vi "TCP设备参数设置.vi"(8 "布尔文本.文本":string, 9 "section (optional)":string, 10 "监测项描述":string) -> (2 "布尔":bool=TRUE, 3 "输出簇":T1)   [LabVIEW 2016, in "环境动力监测库.lvlib"]
uses:
  <vilib>/Utility/miscctls.llb/LVPointTypeDef.ctl
  <vilib>/Utility/config.llb/NI_LVConfig.lvlib
panel:
  in  "Port:":string
  in  "data bits":u64=8 caption="数据比特" min=5 max=8 step=1
  in  "波特率":u64=19200
  in  "停止位":u16(ring)=10 items=["1.0"=10, "1.5"=15, "2.0"=20]
  in  "奇偶校验":u16(ring) items=["None", "Odd", "Even", "Mark", "Space"]
  in  "传感器型号:":string(combo)
  in  "输入簇":T1
  in  "站号":u64
  in  "返回":bool
  in  "增加":bool
  in  "IP address:":string
  in  "监测项描述:":string
  # "基本设置"
  # "如:红外XX"
  # "传感器选择"
  # "地址选择"
  # "站号配置"
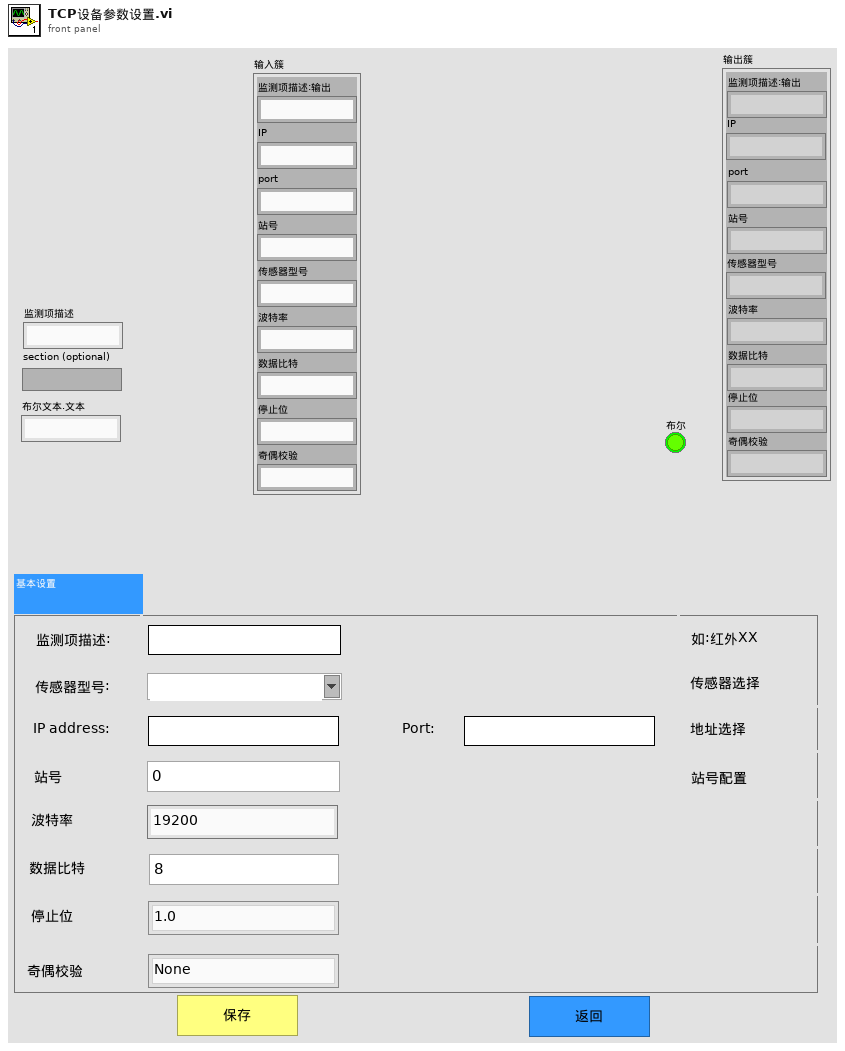
[diagram p1: front panel]
types:
  T1 = cluster{"监测项描述:输出":string, "IP":string, "port":string, "站号":string, "传感器型号":string, "波特率":string, "数据比特":string, "停止位":string, "奇偶校验":string}
  T2 = typedef "LVPointTypeDef.ctl" = cluster{"Horizontal":i16, "Vertical":i16}
  T3 = typedef "NI_LVConfig.lvlib/Config Data RefNum.ctl" = refnum<k1>
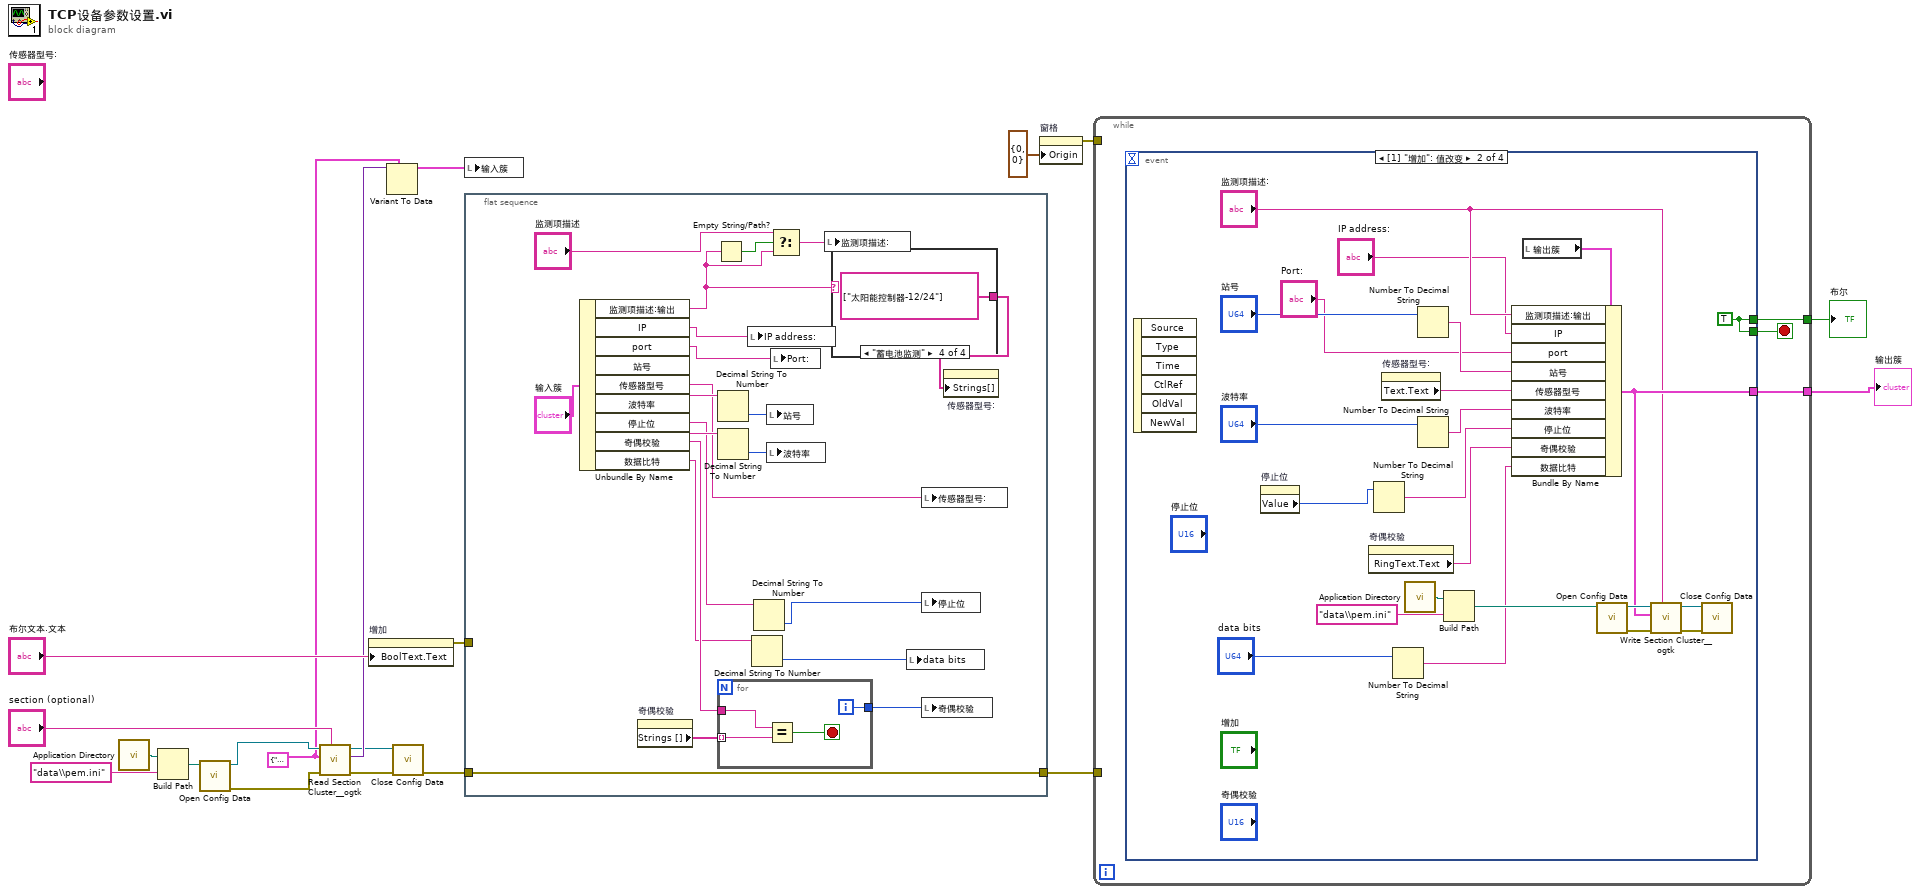
[diagram p0: block diagram]
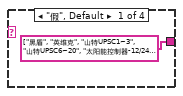
[diagram p2: hidden frame]
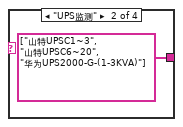
[diagram p3: hidden frame]
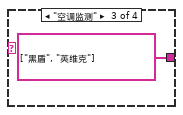
[diagram p4: hidden frame]
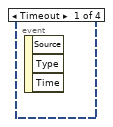
[diagram p5: hidden frame]
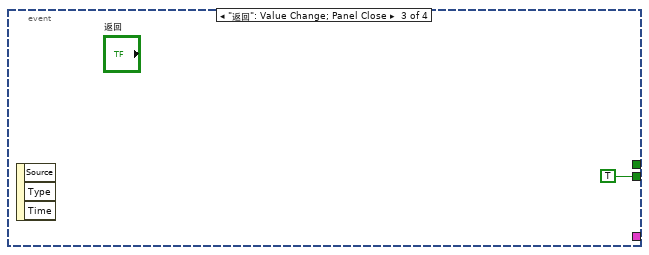
[diagram p6: hidden frame]
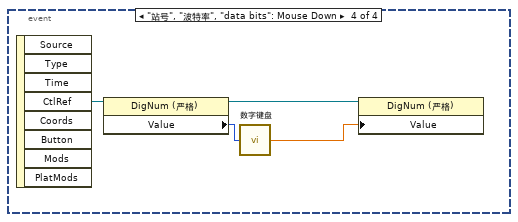
[diagram p7: hidden frame]
diagram:
  w1 = T1 {"监测项描述:输出"="", "IP"="", "port"="", "站号"="", "传感器型号"="", "波特率"="", "数据比特"="", "停止位"="", "奇偶校验"=""} ("数据")
  n1 = call <vilib>:"Application Directory.vi"() -> ("Application Directory"=w12:path)
  n2 = Build Path(base path=w12, name or relative path="data\\pem.ini" ("名称或相对路径")) -> (appended path=w13:path)
  n3 = call <vilib>:"Open Config Data.vi"("configuration file path"=w13) -> ("error out"=w14:errorcluster, "refnum"=w15:T3)  [unwired: 8 in, 1 out]
  n4 = call <userlib>:"Read Section Cluster__ogtk.vi"("section (optional)"="section (optional)", "error in (no error)"=w14, "Section Formatted Cluster Type"=w1, "refnum"=w15) -> ("error out"=w6:errorcluster, "Section Formatted Cluster"=w9:variant, "dup refnum"=w7:T3)  [unwired: 3 in, 2 out]
  n5 = property on="增加" class="Bool"("BoolText.Text"="布尔文本.文本") -> (error out=w5:errorcluster)  [unwired: 2 in, 1 out]
  n6 = Variant To Data(type=w1, Variant=w9) -> (data=w8:T1)  [unwired: 1 in, 1 out]
  n7 = call <vilib>:"Close Config Data.vi"("error in (no error)"=w6, "refnum"=w7) -> ("error out"=w4:errorcluster)  [unwired: 8 in, 1 out]
  n8 = local write "输入簇"(w8) -> ()
  n9 = flat-sequence {
    tunnel: w5 -> [_]
    tunnel: w4 -> [w38]
    tunnel: [w38] -> w3
    frame #0 {
      n10 = Unbundle By Name("输入簇") -> ("监测项描述:输出"=w21:string, "IP"=w24:string, "port"=w23:string, "站号"=w39:string, "传感器型号"=w22:string, "波特率"=w32:string, "停止位"=w28:string, "奇偶校验"=w29:string, "数据比特"=w26:string)
      n11 = property on="奇偶校验" class="Ring (严格)"() -> ("Strings []"=w30:string[])  [unwired: 2 in, 2 out]
      n12 = Empty String/Path?(string/path=w21) -> (empty?=w37:bool)
      n13 = Decimal String To Number(string=w39) -> (number=w34:i32)  [unwired: 2 in, 1 out]
      n14 = Decimal String To Number(string=w32) -> (number=w33:i32)  [unwired: 2 in, 1 out]
      n15 = for {
        tunnel: w29 -> [w48]
        tunnel: [w46] -> w31
        tunnel: w30 -> [w45] mode=indexing
        i -> [w46]
        stop <- w47 stop-if-true
        n16 = Equal?(x=w48, y=w45) -> (x = y?=w47:bool)
      }
      n17 = local write "IP address:"(w24) -> ()
      n18 = Decimal String To Number(string=w26) -> (number=w25:i32)  [unwired: 2 in, 1 out]
      n19 = Decimal String To Number(string=w28) -> (number=w27:i32)  [unwired: 2 in, 1 out]
      n20 = local write "站号"(w34) -> ()
      n21 = local write "波特率"(w33) -> ()
      n22 = Select(t="监测项描述", s=w37, f=w21) -> (s? t:f=w35:string)
      n23 = local write "Port:"(w23) -> ()
      n24 = local write "监测项描述:"(w35) -> ()
      n25 = case shown="\"蓄电池监测\"" w21 {
        tunnel: [string[] ["黑盾", "英维克", "山特UPSC1~3", "山特UPSC6~20", "太阳能控制器-12/24", "华为UPS2000-G-(1-3KVA)"] ("字符串[]") string[] ["山特UPSC1~3", "山特UPSC6~20", "华为UPS2000-G-(1-3KVA)"] ("字符串[]") string[] ["黑盾", "英维克"] ("字符串[]") string[] ["太阳能控制器-12/24"] ("字符串[]")] -> w20
        frame "假", Default {
        }
        frame "UPS监测" {
        }
        frame "空调监测" {
        }
        frame "蓄电池监测" {
        }
      }
      n26 = local write "data bits"(w25) -> ()
      n27 = local write "传感器型号:"(w22) -> ()
      n28 = local write "停止位"(w27) -> ()
      n29 = local write "奇偶校验"(w31) -> ()
      n30 = property on="传感器型号:" class="CmbBox"("Strings[]"=w20) -> ()  [unwired: 2 in, 2 out]
    }
  }
  n31 = property on="窗格" class="Pane"("Origin"=T2 {"Horizontal"=0, "Vertical"=0} ("原点")) -> (error out=w19:errorcluster)  [unwired: 2 in, 1 out]
  n32 = while {
    tunnel: w19 -> [_]
    tunnel: [w51] -> w2
    tunnel: [w49] -> w17
    tunnel: w3 -> [_]
    stop <- w50 stop-if-true
    n33 = event shown="[1] \"增加\": 值改变" {
      selector: _ -> [_ _ _ _]
      dyn-events: _ -> [_ _ _ _]
      timeout: _ -> [_ _ _ _]
      tunnel: [_ w67 _ _] -> w51
      tunnel: [_ w66 TRUE _] -> w50
      tunnel: [_ w66 _ _] -> w49
      event Timeout {
        n34 = event-data() -> ()  [unwired: 1 in, 3 out]
      }
      event "增加": Value Change {
        w66 = TRUE
        n35 = event-data() -> ()  [unwired: 1 in, 6 out]
        n36 = property on="停止位" class="Ring (严格)"() -> ("Value"=w59:u16)  [unwired: 2 in, 2 out]
        n37 = property on="奇偶校验" class="Ring (严格)"() -> ("RingText.Text"=w60:string)  [unwired: 2 in, 2 out]
        n38 = Number To Decimal String(number=w59) -> (decimal integer string=w58:string)  [unwired: 1 in]
        n39 = property on="传感器型号:" class="CmbBox"() -> ("Text.Text"=w63:string)  [unwired: 2 in, 2 out]
        n40 = Number To Decimal String(number="data bits") -> (decimal integer string=w57:string)  [unwired: 1 in]
        n41 = call <vilib>:"Application Directory.vi"() -> ("Application Directory"=w71:path)
        n42 = Number To Decimal String(number="站号") -> (decimal integer string=w65:string)  [unwired: 1 in]
        n43 = Number To Decimal String(number="波特率") -> (decimal integer string=w61:string)  [unwired: 1 in]
        n44 = Build Path(base path=w71, name or relative path="data\\pem.ini" ("名称或相对路径")) -> (appended path=w72:path)
        n45 = local read "输出簇"() -> (w52:T1)
        n46 = Bundle By Name(cluster=w52, "监测项描述:输出"="监测项描述:", "IP"="IP address:", "port"="Port:", "站号"=w65, "传感器型号"=w63, "波特率"=w61, "停止位"=w58, "奇偶校验"=w60, "数据比特"=w57) -> (w67:T1)
        n47 = call <vilib>:"Open Config Data.vi"("configuration file path"=w72) -> ("error out"=w73:errorcluster, "refnum"=w74:T3)  [unwired: 8 in, 1 out]
        n48 = call <userlib>:"Write Section Cluster__ogtk.vi"("section (optional)"="监测项描述:", "error in (no error)"=w73, "Section Formatted Cluster"=w67, "refnum"=w74) -> ("error out"=w68:errorcluster, "dup refnum"=w69:T3)  [unwired: 6 in]
        n49 = call <vilib>:"Close Config Data.vi"("error in (no error)"=w68, "refnum"=w69) -> ()  [unwired: 8 in, 2 out]
      }
      event "返回": Value Change; Panel Close {
        n50 = event-data() -> ()  [unwired: 1 in, 3 out]
      }
      event "站号", "波特率", "data bits": Mouse Down {
        n51 = event-data() -> ("CtlRef"=w79:refnum<vi>)  [unwired: 1 in, 7 out]
        n52 = property class="DigNum (严格)"(reference=w79) -> (reference out=w77:refnum<vi>, "Value"=w78:u64)  [unwired: 1 in, 1 out]
        n53 = call "数字键盘.vi"("OldNumber"=w78) -> ("NewNumber"=w76:sgl)
        n54 = property class="DigNum (严格)"(reference=w77, "Value"=w76) -> ()  [unwired: 1 in, 2 out]
      }
    }
  }
  "输出簇" <- w2
  "布尔" <- w17
